vi "题目6.vi"   [LabVIEW 2017]
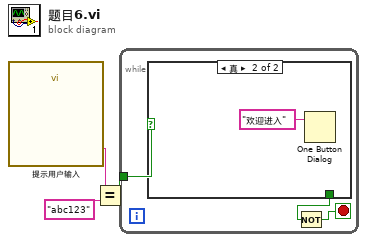
[diagram p0: block diagram]
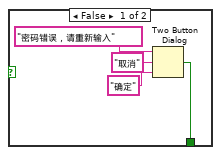
[diagram p2: hidden frame]
diagram:
  n1 = call "提示用户输入"() -> ("请输入秘码"=w1:string)  [unwired: 17 in, 2 out]
  n2 = Equal?(x=w1, y="abc123") -> (x = y?=w2:bool)
  n3 = while {
    tunnel: w2 -> [w6]
    stop <- w4 stop-if-true
    n4 = case shown="真" w6 {
      tunnel: [w9 _] -> w5
      frame False {
        n5 = Two Button Dialog(message="密码错误，请重新输入" ("消息"), 1:"确定" ("F按钮名称（“取消”）"), 2:"取消" ("T按钮名称（“确定”）")) -> (T button?=w9:bool)
      }
      frame True {
        n6 = One Button Dialog(message="欢迎进入" ("消息")) -> ()  [unwired: 1 in, 1 out]
      }
    }
    n7 = Not(x=w5) -> (.not. x?=w4:bool)
  }
